vi "LM model function and gradient.vi"(3 "output control":T1, 4 "data":variant, 5 "X":dbl[](array[numeric]), 6 "a":dbl[](array[numeric])) -> (0 "error out":errorcluster, 1 "f'(X,a)":dbl[][](array[numeric]), 2 "f(X,a)":dbl[](array[numeric]))   [LabVIEW 2019]
doc: "This template is the starting point for creating a model function to be passed to the Nonlinear Curve Fit.vi."
uses:
  <vilib>/gmath/NumericalOptimization/LM_output select.ctl
  <vilib>/gmath/NI_Gmath.lvlib
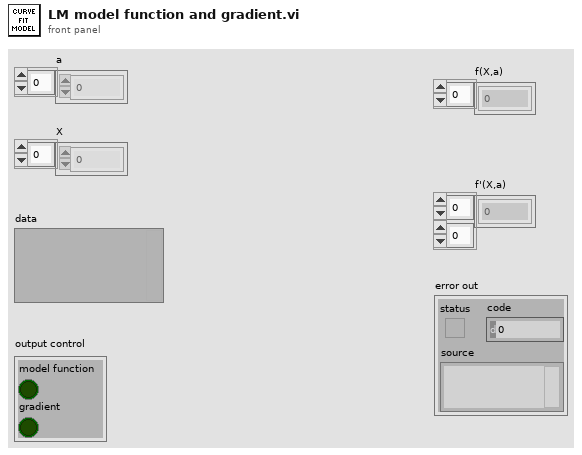
[diagram p1: front panel]
types:
  T1 = typedef "NI_Gmath.lvlib/LM_output select.ctl" = cluster{"model function":bool, "gradient":bool}
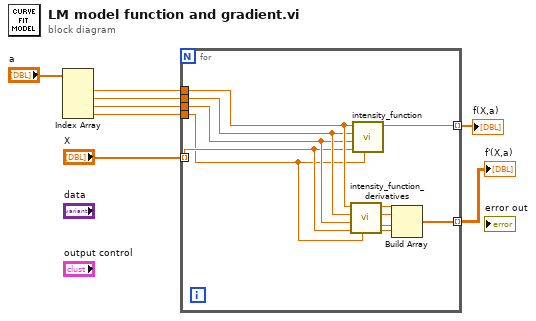
[diagram p0: block diagram]
diagram:
  n1 = Index Array(array="a") -> (element #1=w6:dbl, element #2=w5:dbl, element #3=w4:dbl, element #4=w3:dbl)  [unwired: 4 in]
  n2 = for {
    tunnel: "X" -> [w15] mode=indexing
    tunnel: w6 -> [w18]
    tunnel: w5 -> [w17]
    tunnel: w4 -> [w16]
    tunnel: w3 -> [w14]
    tunnel: [w19] -> w2 mode=indexing
    tunnel: [w9] -> w1 mode=indexing
    n3 = call "intensity_function_derivatives.vi"("theta_min"=w14, "theta"=w15, "C"=w16, "B"=w17, "A"=w18) -> ("dThetaMin"=w12:dbl, "dC"=w11:dbl, "dB"=w10:dbl, "dA"=w13:dbl)  [unwired: 3 in]
    n4 = call "intensity_function.vi"("theta_min"=w14, "theta"=w15, "C"=w16, "B"=w17, "A"=w18) -> ("output variable"=w19:dbl)  [unwired: 6 in]
    n5 = Build Array(w13, w10, w11, w12) -> (w9:dbl[])
  }
  "f(X,a)" <- w2
  "f'(X,a)" <- w1
